vi "myRIO_BRig_RT_TCP.vi"(0 "input_hTCP":refnum<k5>, 1 "input_AI1":i16, 2 "input_AI0":i16, 3 "input_I_connected_TCP":bool, 5 "input_index":i32, 7 "input_iBlock":u16, 9 "input_iTrial":u16, 11 "input_error":errorcluster, 12 "input_iEvent":u16, 13 "input_iState":T1) -> (4 "output_hTCP":refnum<k5>, 15 "output_error":errorcluster)   [LabVIEW 2014]
uses:
  myRIO_BRig_RT__Case_Exp_stateList.ctl
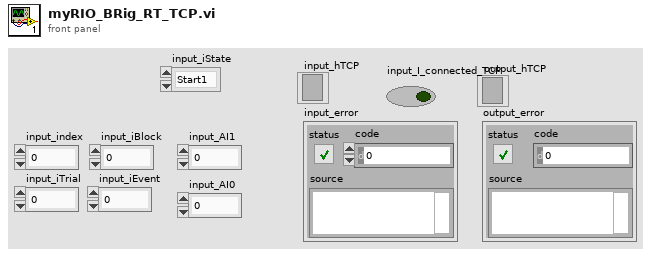
[diagram p1: front panel]
types:
  T1 = typedef "myRIO_BRig_RT__Case_Exp_stateList.ctl" = enum16{"Start1", "Start2", "Start3", "saveSettings1", "saveSettings2", "saveSettings3", "saveSettings4_LC_ENL", "saveSettings5_LC_Cue", "saveSettings6_LC_Other", "setSettings_Audio", "setSettings_Laser", "initBlock_pre", "initBlock", "initBlock2", "initBlock_post", "initTrial_pre", "initTrial", "initTrial2", "initTrial3", "initTrial4", "initTrial_LC_ENL1", "initTrial_LC_Cue1", "initTrial_LC_Sel", "initTrial_post", "ENL1_pre", "ENL1", "ENL1_post", "ENL1Penalty_pre", "ENL1Penalty", "ENL2_pre", "ENL2", "ENL2Penalty_pre", "ENL2Penalty", "Cue1_pre", "Cue1", "Cue1_post", "Cue1Penalty_pre", "Cue1Penalty", "Cue2_pre", "Cue2", "Cue2Penalty_pre", "Cue2Penalty", "Selection_pre", "Selection", "Select_post", "SelectReward_pre", "SelectReward", "SelectRewardPost_pre", "SelectRewardPost", "SelectWrong_pre", "SelectWrong", "SelectWrong_post", "SelectTimeout_pre", "SelectTimeout", "SelectTimeout_post", "endTrial_pre", "endTrial1", "endTrial2", "endTrial3", "endTrial_post", "endBlock_pre", "endBlock", "endBlock_post", "endExp", "commConnect", "commUpload_pre", "commUpload_dataBlock", "commUpload_dataCurrent", "commUpload_dataExp", "commUpload_dataLC", "commUpload_dataTrial", "commUpload_post", "saveData_pre", "saveData_dataBlock", "saveData_dataCurrent", "saveData_dataExp", "saveData_dataLC", "saveData_dataTrial", "saveData_post", "empty_endBlock1", "empty_endBlock2", "empty_endTrial1", "empty_endTrial2", "empty_endTrial3", "empty_endTrial4", "empty_endTrial5"}
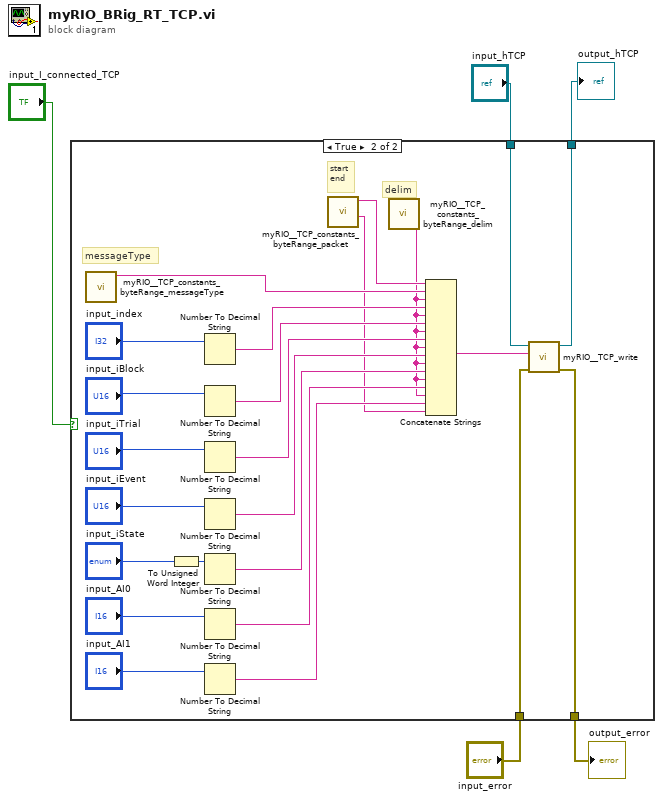
[diagram p0: block diagram]
diagram:
  n1 = case shown="True" "input_I_connected_TCP" {
    tunnel: "input_hTCP" -> [w7 w12]
    tunnel: "input_error" -> [w6 w11]
    tunnel: [w7 w10] -> w3
    tunnel: [w6 w9] -> w2
    frame False {
    }
    frame True {
      # "messageType"
      # "start\nend"
      # "delim"
      n2 = call "myRIO__TCP_constants_byteRange_messageType.vi"() -> ("output_Trial_char"=w22:string)  [unwired: 6 in, 5 out]
      n3 = To Unsigned Word Integer(number="input_iState") -> (unsigned 16bit integer=w30:u16)
      n4 = Number To Decimal String(number="input_index") -> (decimal integer string=w21:string)  [unwired: 1 in]
      n5 = Number To Decimal String(number="input_iBlock") -> (decimal integer string=w20:string)  [unwired: 1 in]
      n6 = Number To Decimal String(number="input_iTrial") -> (decimal integer string=w19:string)  [unwired: 1 in]
      n7 = Number To Decimal String(number="input_iEvent") -> (decimal integer string=w18:string)  [unwired: 1 in]
      n8 = Number To Decimal String(number=w30) -> (decimal integer string=w17:string)  [unwired: 1 in]
      n9 = Number To Decimal String(number="input_AI0") -> (decimal integer string=w16:string)  [unwired: 1 in]
      n10 = Number To Decimal String(number="input_AI1") -> (decimal integer string=w15:string)  [unwired: 1 in]
      n11 = call "myRIO__TCP_constants_byteRange_packet.vi"() -> ("output_end_char"=w8:string, "output_start_char"=w23:string)  [unwired: 8 in, 2 out]
      n12 = call "myRIO__TCP_constants_byteRange_delim.vi"() -> ("output_delim_char"=w14:string)  [unwired: 10 in, 1 out]
      n13 = Concatenate Strings(w23, w22, w14, w21, w14, w20, w14, w19, w14, w18, w14, w17, w14, w16, w14, w15, w8) -> (w13:string)
      n14 = call "myRIO__TCP_write.vi"("input_error"=w11, "input_packet"=w13, "input_hTCP"=w12) -> ("output_error"=w9:errorcluster, "output_hTCP"=w10:refnum<k5>)  [unwired: 6 in, 1 out]
    }
  }
  "output_hTCP" <- w3
  "output_error" <- w2
